vi "set extio settings.vi"(8 "error in (no error)":errorcluster, 10 "extio_settings":T1, 11 "id":i32) -> (0 "error out":errorcluster, 3 "function return":i32)   [LabVIEW 2012, in "libximc.lvlib"]
doc: "result_t XIMC_API set_extio_settings (device_t id, const extio_settings_t* extio_settings);"
uses:
  libximc.lvlib
  libximc.dll
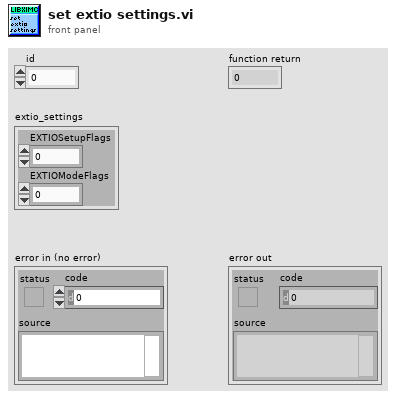
[diagram p1: front panel]
types:
  T1 = cluster{"EXTIOSetupFlags":u32, "EXTIOModeFlags":u32}
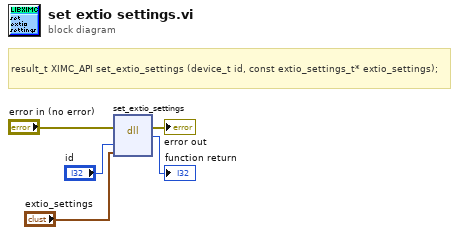
[diagram p0: block diagram]
diagram:
  # "result_t XIMC_API set_extio_settings (device_t id, const extio_settings_t* extio_settings);"
  n1 = dll-call lib="E:/labview-2.12.1-Labview_12.0/ximcLVx32/libximc.*" fn="set_extio_settings"(error in="error in (no error)", "id"="id", "extio_settings"="extio_settings") -> (error out=→"error out":errorcluster, →"function return":i32)  [unwired: 4 in, 1 out]
